vi "未命名 4.vi"() -> ()   [LabVIEW 2020, in "PCANBasic.lvlib"]
uses:
  <userlib>/PCANBasic/PCANBasic.lvlib
panel:
  out "文本下拉列表":u16(ring) items=["xxx", "PCAN_DEVICE_ID", "PCAN_5VOLTS_POWER", "PCAN_RECEIVE_EVENT", "PCAN_MESSAGE_FILTER", "PCAN_API_VERSION", "PCAN_CHANNEL_VERSION", "PCAN_BUSOFF_AUTORESET", "PCAN_LISTEN_ONLY", "PCAN_LOG_LOCATION", "PCAN_LOG_STATUS", "PCAN_LOG_CONFIGURE", "PCAN_LOG_TEXT", "PCAN_CHANNEL_CONDITION", "PCAN_HARDWARE_NAME", "PCAN_RECEIVE_STATUS", "PCAN_CONTROLLER_NUMBER", "PCAN_TRACE_LOCATION", "PCAN_TRACE_STATUS", "PCAN_TRACE_SIZE", "PCAN_TRACE_CONFIGURE", "PCAN_CHANNEL_IDENTIFYING", "PCAN_CHANNEL_FEATURES", "PCAN_BITRATE_ADAPTING", "PCAN_BITRATE_INFO", "PCAN_BITRATE_INFO_FD", "PCAN_BUSSPEED_NOMINAL", "PCAN_BUSSPEED_DATA", "PCAN_IP_ADDRESS", "PCAN_LAN_SERVICE_STATUS", "PCAN_ALLOW_STATUS_FRAMES", "PCAN_ALLOW_RTR_FRAMES", "PCAN_ALLOW_ERROR_FRAMES", "PCAN_INTERFRAME_DELAY", "PCAN_ACCEPTANCE_FILTER_11BIT", "PCAN_ACCEPTANCE_FILTER_29BIT", "PCAN_IO_DIGITAL_CONFIGURATION", "PCAN_IO_DIGITAL_VALUE", "PCAN_IO_DIGITAL_SET", "PCAN_IO_DIGITAL_CLEAR", "PCAN_IO_ANALOG_VALUE", "PCAN_FIRMWARE_VERSION", "PCAN_ATTACHED_CHANNELS_COUNT", "PCAN_ATTACHED_CHANNELS"]
  out "string array":string[](array[string]) caption="字符串数组"
  out "结果字符串":string
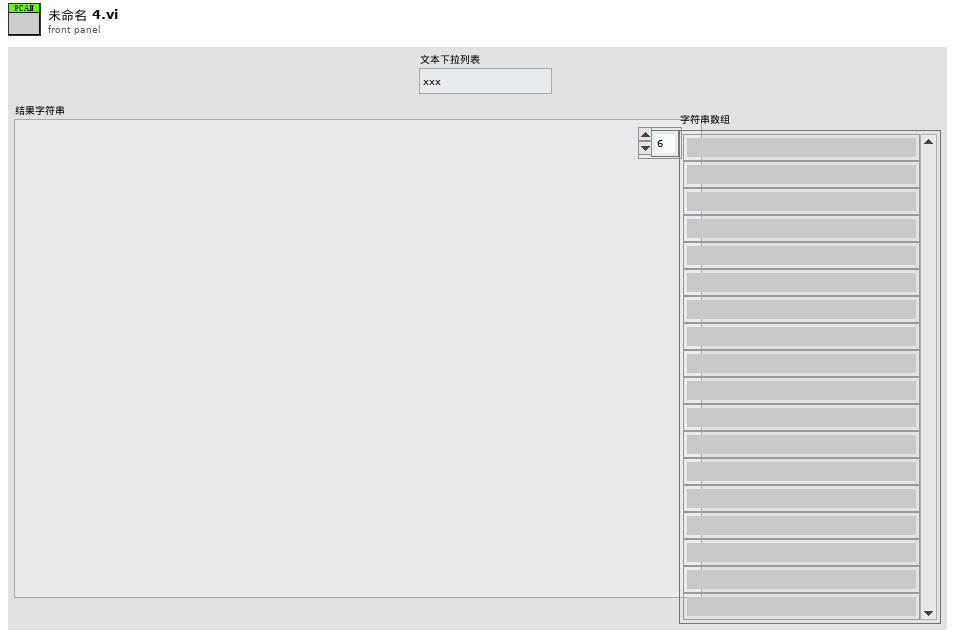
[diagram p1: front panel]
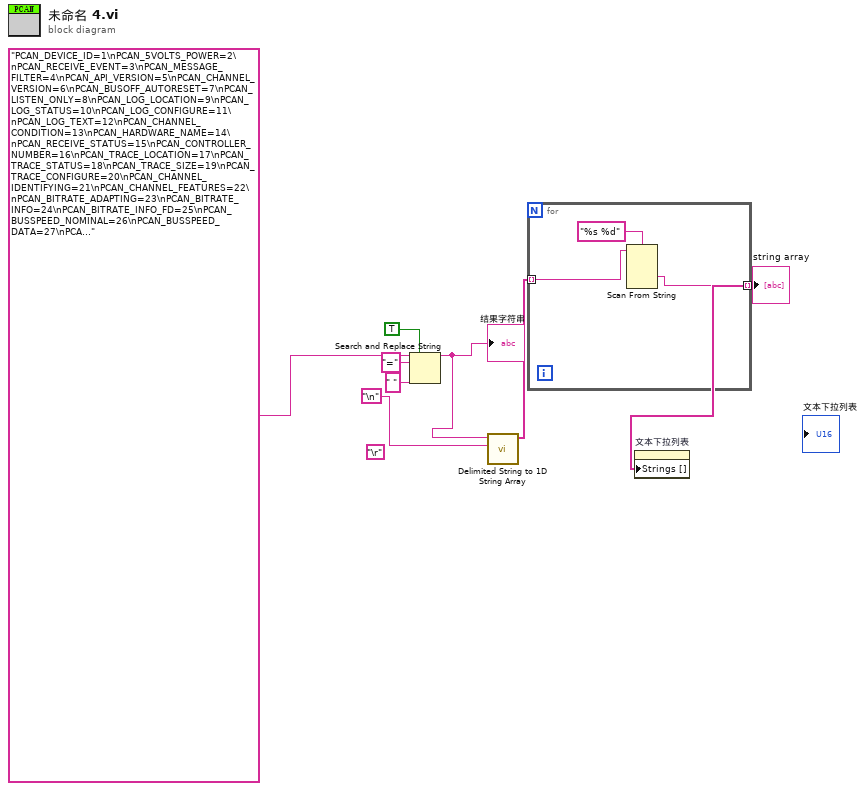
[diagram p0: block diagram]
diagram:
  (unwired) "\r"
  n1 = Search and Replace String(replace all?=TRUE ("替换全部？(F)"), input string="PCAN_DEVICE_ID=1\nPCAN_5VOLTS_POWER=2\nPCAN_RECEIVE_EVENT=3\nPCAN_MESSAGE_FILTER=4\nPCAN_API_VERSION=5\nPCAN_CHANNEL_VERSION=6\nPCAN_BUSOFF_AUTORESET=7\nPCAN_LISTEN_ONLY=8\nPCAN_LOG_LOCATION=9\nPCAN_LOG_STATUS=10\nPCAN_LOG_CONFIGURE=11\nPCAN_LOG_TEXT=12\nPCAN_CHANNEL_CONDITION=13\nPCAN_HARDWARE_NAME=14\nPCAN_RECEIVE_STATUS=15\nPCAN_CONTROLLER_NUMBER=16\nPCAN_TRACE_LOCATION=17\nPCAN_TRACE_STATUS=18\nPCAN_TRACE_SIZE=19\nPCAN_TRACE_CONFIGURE=20\nPCAN_CHANNEL_IDENTIFYING=21\nPCAN_CHANNEL_FEATURES=22\nPCAN_BITRATE_ADAPTING=23\nPCAN_BITRATE_INFO=24\nPCAN_BITRATE_INFO_FD=25\nPCAN_BUSSPEED_NOMINAL=26\nPCAN_BUSSPEED_DATA=27\nPCAN_IP_ADDRESS=28\nPCAN_LAN_SERVICE_STATUS=29\nPCAN_ALLOW_STATUS_FRAMES=30\nPCAN_ALLOW_RTR_FRAMES=31\nPCAN_ALLOW_ERROR_FRAMES=32\nPCAN_INTERFRAME_DELAY=33\nPCAN_ACCEPTANCE_FILTER_11BIT=34\nPCAN_ACCEPTANCE_FILTER_29BIT=35\nPCAN_IO_DIGITAL_CONFIGURATION=36\nPCAN_IO_DIGITAL_VALUE=37\nPCAN_IO_DIGITAL_SET=38\nPCAN_IO_DIGITAL_CLEAR=39\nPCAN_IO_ANALOG_VALUE=40\nPCAN_FIRMWARE_VERSION=41\nPCAN_ATTACHED_CHANNELS_COUNT=42\nPCAN_ATTACHED_CHANNELS=43", search string="=" ("搜索字符串"), replace string=" " ("替换字符串(\"\")")) -> (result string=w7:string)  [unwired: 4 in, 3 out]
  "结果字符串" <- w7
  n2 = call <vilib>:"Delimited String to 1D String Array.vi"("delimiter"="\n", "delimited string"=w7) -> ("string array"=w3:string[])  [unwired: 9 in]
  n3 = for {
    tunnel: w3 -> [w10] mode=indexing
    tunnel: [w9] -> w2 mode=indexing
    n4 = Scan From String(format string="%s %d" ("格式字符串"), input string=w10) -> (output 1=w9:string)  [unwired: 5 in, 3 out]
  }
  "string array" <- w2
  n5 = property on="文本下拉列表" class="Ring (严格)"("Strings []"=w2) -> ()  [unwired: 2 in, 2 out]
